vi "MT Set Axis Position Dec.vi"(10 "Value":i32, 11 "AObj":u16) -> (3 "function return":i32)   [LabVIEW 2014, in "MT_API.lvlib"]
doc: "MT_API INT32 __stdcall MT_Set_Axis_Position_Dec(WORD AObj,INT32 Value);"
uses:
  MT_API.lvlib
  MT_API.dll
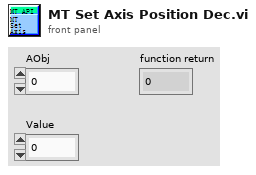
[diagram p1: front panel]
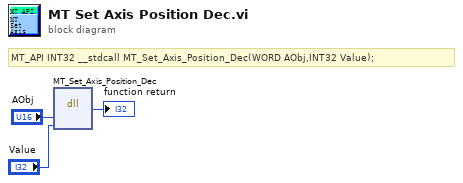
[diagram p0: block diagram]
diagram:
  # "MT_API INT32 __stdcall MT_Set_Axis_Position_Dec(WORD AObj,INT32 Value);"
  n1 = dll-call lib="E:/Projects/LabView/MT_API/MT_API.*" fn="MT_Set_Axis_Position_Dec"("AObj"="AObj", "Value"="Value") -> (→"function return":i32)  [unwired: 5 in, 2 out]
